vi "GetUnit.vi"(8 "error in":errorcluster, 11 "Measure in":refnum<class "Measure.lvclass">) -> (0 "error out":errorcluster, 2 "Unit":T1, 3 "Measure out":refnum<class "Measure.lvclass">)   [LabVIEW 2021, in "ProligentXMLGenerator.lvlib" / "Measure.lvclass"]
doc: "Defines the name of the unit of the measure value (Ex: kilometer). When a unit symbol is provided, the unit name becomes required.\nDefines the symbol of the unit for the measure value (ex: km). When a unit name is provided, the unit symbol becomes required.\n\nUnit Name vaule is restricted to 30 characters and Unit Symbol is restricted to 20 characters."
uses:
  Measure.lvclass
  Measure.lvclass/Measure.ctl
  Unit.ctl
  Base/NonEmptyString_20/NonEmptyString_20.lvclass
  Base/NonEmptyString_30/NonEmptyString_30.lvclass
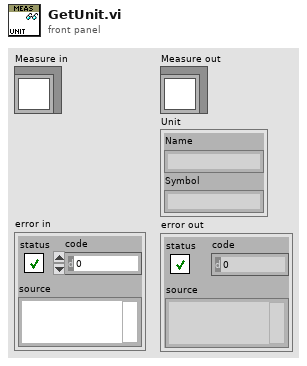
[diagram p1: front panel]
types:
  T1 = typedef "ProligentXMLGenerator.lvlib/Measure.lvclass/Unit.ctl" = cluster{"Name":string, "Symbol":string}
  T2 = typedef "ProligentXMLGenerator.lvlib/Measure.lvclass/Data.ctl" = cluster{"Name":string, "Type":refnum<class "MeasureKind.lvclass">, "Precision":refnum<class "UnsignedByte.lvclass">, "Limit":refnum<class "MeasureLimit.lvclass">, "Characteristics":refnum<class "Characteristic.lvclass">[], "FailureReferences":refnum<class "FailureReference.lvclass">[], "CustomData":refnum<class "CustomData.lvclass">, "MeasureId":refnum<class "Guid.lvclass">, "MeasureTime":refnum<class "DateTime.lvclass">, "Comments":refnum<class "NonNullableString_TruncateAt_255.lvclass">, "Unit":refnum<class "NonEmptyString_30.lvclass">, "Symbol":refnum<class "NonEmptyString_20.lvclass">, "MeasureExecutionStatus":refnum<class "ExecutionStatus.lvclass">}
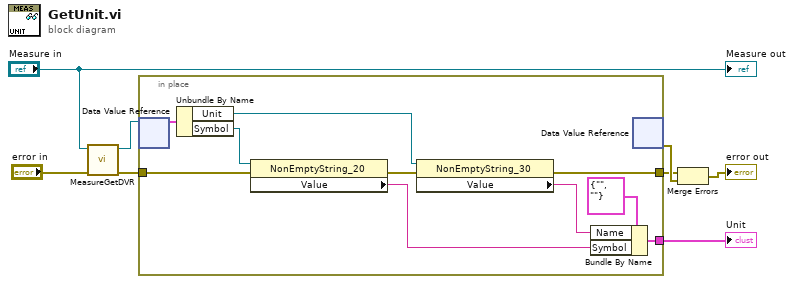
[diagram p0: block diagram]
diagram:
  n1 = call "MeasureGetDVR.vi"("error in"="error in", "Measure"="Measure in") -> ("error out"=w3:errorcluster, "DVRReference"=w7:refnum<data-value>)  [unwired: 8 in]
  n2 = in-place "In Place Element Structure" {
    in-place-border: w3 -> [w14]
    in-place-border: [w16] -> w2
    in-place-border: [w9] -> w1
    n3 = in-place-dvr #1(w7) -> (w18:T2)  [unwired: 1 out]
    n4 = Unbundle By Name(w18) -> ("Unit"=w17:refnum<class "NonEmptyString_30.lvclass">, "Symbol"=w15:refnum<class "NonEmptyString_20.lvclass">)
    n5 = property on="Property Node" class="NonEmptyString_20"(reference=w15, error in=w14) -> (error out=w13:errorcluster, "Value"=w12:string)  [unwired: 1 out]
    n6 = property on="Property Node" class="NonEmptyString_30"(reference=w17, error in=w13) -> (error out=w16:errorcluster, "Value"=w10:string)  [unwired: 1 out]
    n7 = Bundle By Name(cluster=T1 {"Name"="", "Symbol"=""} ("MeasureTime"), "Name"=w10, "Symbol"=w12) -> (w9:T1)
    n8 = in-place-dvr #1() -> (w8:errorcluster)  [unwired: 1 in, 1 out]
  }
  "Unit" <- w1
  n9 = Merge Errors(w2, w8) -> (→"error out":errorcluster)
  "Measure out" <- "Measure in"
